vi "Global.vi"() -> ()   [LabVIEW 2011]
panel:
  in  "Numeric":i32
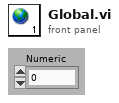
[diagram p1: front panel]
diagram:
